vi "sinx.vi"() -> ()   [LabVIEW 2019]
panel:
  in  "sinx":dbl
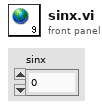
[diagram p1: front panel]
diagram:
